vi "Epoxy_Cycle Execute.vi"(8 "error in (no error)":errorcluster, 10 "Refs In":T2, 11 "Data Cluster In":T1) -> (0 "error out":errorcluster, 2 "Int Lap [s] out":dbl, 3 "Data Cluster Out":T1)   [LabVIEW 2020]
uses:
  controls/CycleTimer.ctl
  controls/Valves Radio.ctl
  controls/UI Data.ctl
  DAQLoop_Typedef.ctl
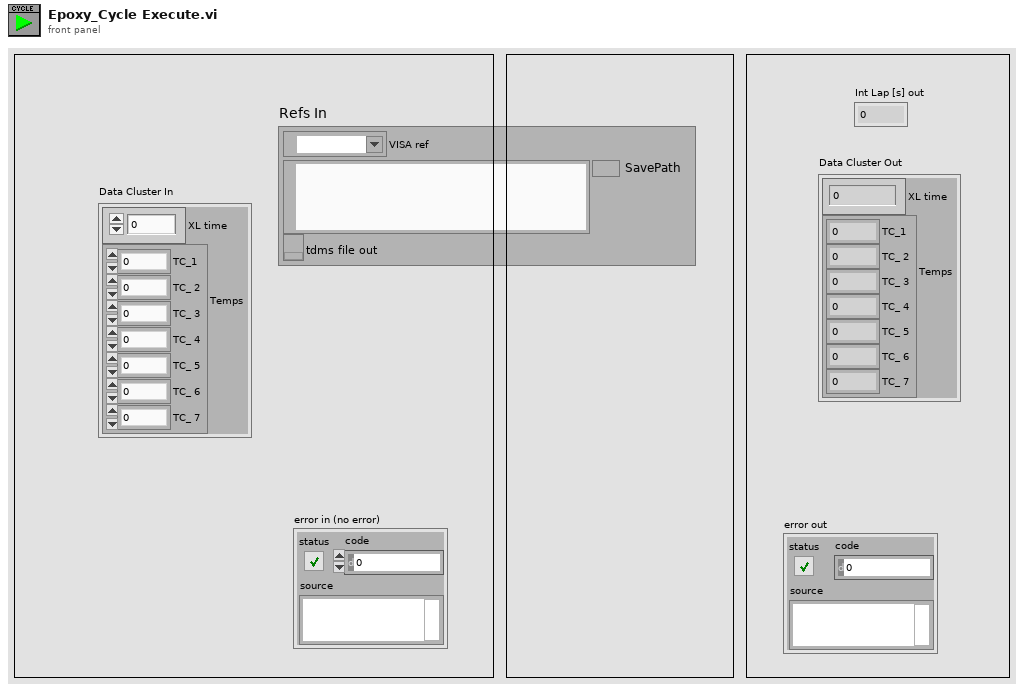
[diagram p1: front panel]
types:
  T1 = typedef "DAQLoop_Typedef.ctl" = cluster{"XL time":dbl, "Temps":cluster{"TC_1":dbl, "TC_ 2":dbl, "TC_ 3":dbl, "TC_ 4":dbl, "TC_ 5":dbl, "TC_ 6":dbl, "TC_ 7":dbl}}
  T2 = typedef "UI Data.ctl" = cluster{"VISA ref":refnum<visa-resource-name>, "SavePath":path, "tdms file out":refnum<k34>}
  T3 = typedef "CycleTimer.ctl" = enum16{"Start Cycle", "StartInterval", "UpdateInterval", "Check"}
  T4 = typedef "Valves Radio.ctl" = enum32{"A", "B"}
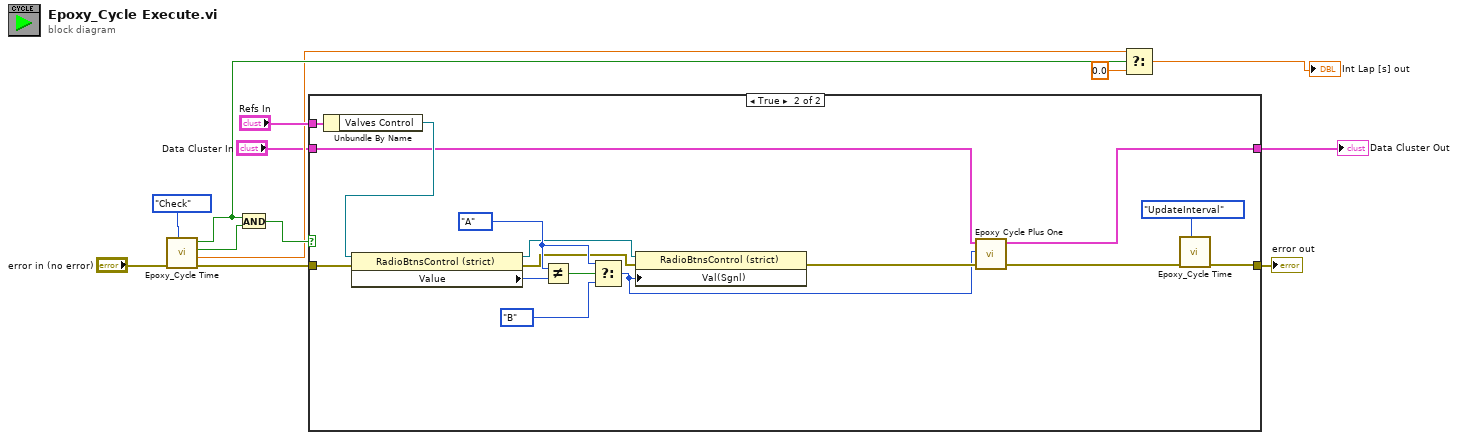
[diagram p0: block diagram]
diagram:
  n1 = call "Epoxy_Cycle Time.vi"("Enum"=CycleTimer."Check", "error in (no error)"="error in (no error)") -> ("error out"=w11:errorcluster, "Int Lap [s]"=w5:dbl, "Cycle done?"=w8:bool, "Running?"=w6:bool)  [unwired: 6 in]
  n2 = And(x=w6, y=w8) -> (x .and. y?=w7:bool)
  n3 = case shown="True" w7 {
    tunnel: w11 -> [w15 w27]
    tunnel: [w15 w31] -> w12
    tunnel: "Refs In" -> [_ w29]
    tunnel: "Data Cluster In" -> [w14 w20]
    tunnel: [w14 w19] -> w1
    frame False {
    }
    frame True {
      w24 = Valves_Radio."A" ("Valves Control")
      n4 = Unbundle By Name(w29) -> ("Valves Control"=w28:refnum<vi>)
      n5 = property class="RadioBtnsControl (strict)"(reference=w28, error in=w27) -> (reference out=w22:refnum<vi>, error out=w21:errorcluster, "Value"=w26:T4)
      n6 = Not Equal?(x=w24, y=w26) -> (x != y?=w25:bool)
      n7 = Select(t=w24, s=w25, f=Valves_Radio."B" ("Valves Control")) -> (s? t:f=w16:T4)
      n8 = property class="RadioBtnsControl (strict)"(reference=w22, error in=w21, "Val(Sgnl)"=w16) -> (error out=w18:errorcluster)  [unwired: 1 out]
      n9 = call "Epoxy Cycle Plus One.vi"("error in (no error)"=w18, "Valves Control"=w16, "Data Cluster In in"=w20) -> ("error out"=w17:errorcluster, "Data Cluster In out"=w19:T1)  [unwired: 7 in]
      n10 = call "Epoxy_Cycle Time.vi"("Enum"=CycleTimer."UpdateInterval", "error in (no error)"=w17) -> ("error out"=w31:errorcluster)  [unwired: 6 in, 3 out]
    }
  }
  "error out" <- w12
  "Data Cluster Out" <- w1
  n11 = Select(t=w5, s=w6, f=0.0) -> (s? t:f=→"Int Lap [s] out":dbl)
